vi "Display.vi"(8 "error in":errorcluster, 11 "Input (String) in":refnum<class "Input (String).lvclass">) -> (0 "error out":errorcluster, 3 "Input (String) out":refnum<class "Input (String).lvclass">)   [LabVIEW 2021, in "Pop-Up.lvlib" / "Input (String).lvclass"]
doc: "This vi will display the input pop up waiting for a type String input from the user\n\n<b>Code Developed By:</b>\nDaniel Coons\nTechnology Service Corporation\n1983 S Liberty Drive\nBloomington, IN 47403\nPhone: 812 558-7100\ndaniel.coons@tsc.com\nwww.tsc.com/atcs"
uses:
  Input (String).lvclass
  C:/Development/Open Source/tsc-pop-up/Popup/Popup.lvclass
  Input (String).lvclass/Input (String).ctl
  Popup/Popup.lvclass/Popup.ctl
  Popup/Data Member Access/Read Theme.vi
  Theme/Theme.lvclass
  Popup/Popup.lvclass
  user32.dll
panel:
  out "header":bool
  out "2D Picture":picture
  in  "OK Button":bool
  out "String":string
  in  "Input":string
  out "Input value out":string
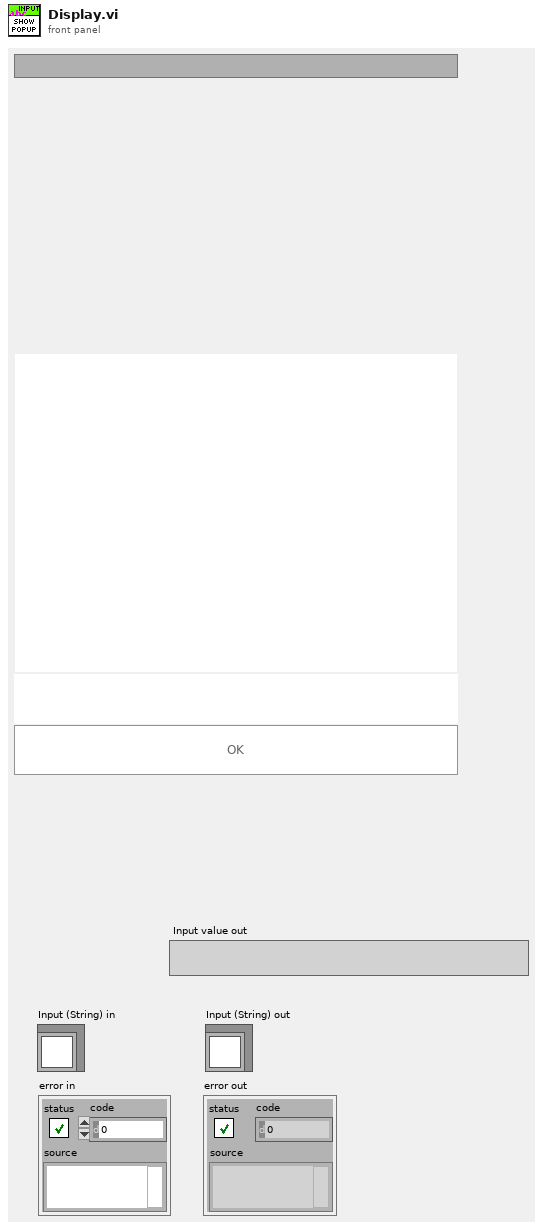
[diagram p1: front panel]
types:
  T1 = typedef "LVPoint32TypeDef.ctl" = cluster{"Horizontal":i32, "Vertical":i32}
  T2 = typedef "LVPositionTypeDef.ctl" = cluster{"Left":i32, "Top":i32}
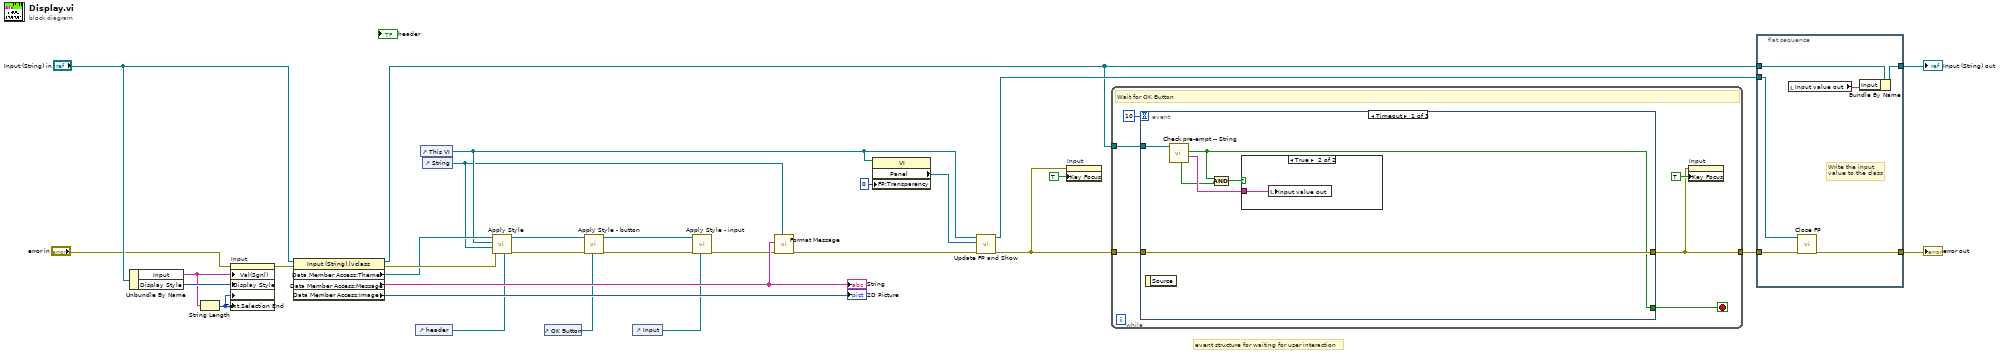
[diagram p0: block diagram]
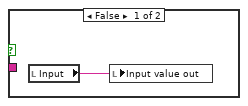
[diagram p2: hidden frame]
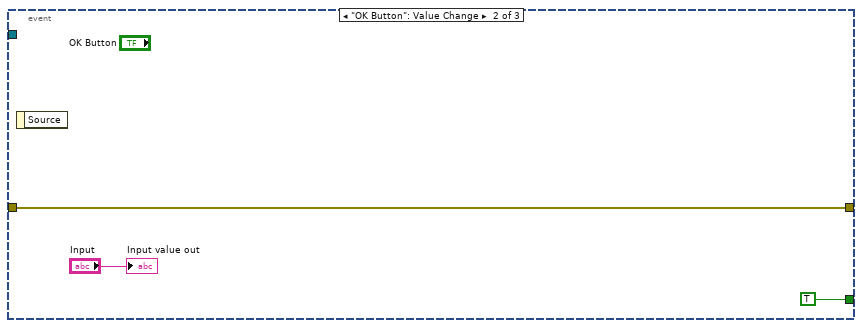
[diagram p3: hidden frame]
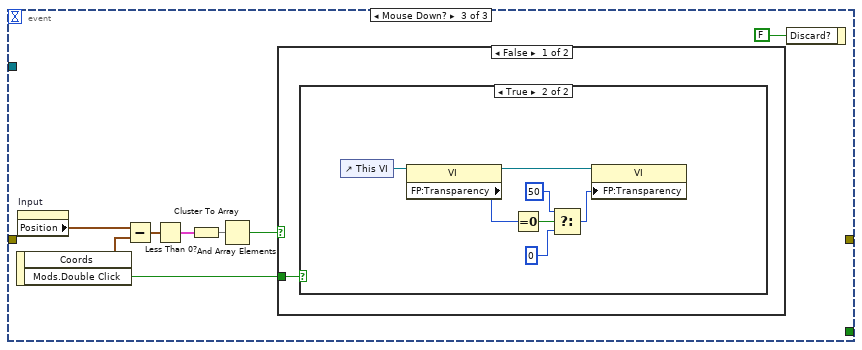
[diagram p4: hidden frame]
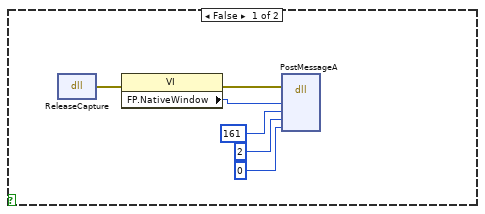
[diagram p5: hidden frame]
diagram:
  # "event structure for waiting for user interaction"
  n1 = Unbundle By Name("Input (String) in") -> ("Input"=w15:string, "Display Style"=w16:u32)
  n2 = String Length(string=w15) -> (length=w14:i32)
  n3 = property on="Input" class="Str"(error in="error in", "Val(Sgnl)"=w15, "Display Style"=w16, "Text.Selection Start"=w14, "Text.Selection End"=w14) -> (error out=w27:errorcluster)  [unwired: 1 in, 1 out]
  n4 = property on="Property Node" class="Input (String).lvclass"(reference="Input (String) in", error in=w27) -> (reference out=w20:refnum<class "Input (String).lvclass">, error out=w26:errorcluster, "Data Member Access:Theme"=w12:refnum<class "Theme.lvclass">, "Data Member Access:Message"=w18:string, "Data Member Access:Image"=→"2D Picture":picture)
  "String" <- w18
  n5 = control-ref of="header"() -> (w9:refnum<vi>)
  n6 = control-ref of="This VI"() -> (w11:refnum<vi>)
  n7 = control-ref of="String"() -> (w10:refnum<vi>)
  n8 = call "Apply Style.vi"("header ref"=w9, "error in"=w26, "message ref"=w10, "pop up ref"=w11, "Theme in"=w12) -> ("error out"=w13:errorcluster, "Theme out"=w5:refnum<class "Theme.lvclass">)  [unwired: 5 in]
  n9 = control-ref of="OK Button"() -> (w4:refnum<vi>)
  n10 = call "Apply Style - button.vi"("button ref"=w4, "error in"=w13, "Theme in"=w5) -> ("error out"=w8:errorcluster, "Theme out"=w6:refnum<class "Theme.lvclass">)  [unwired: 7 in]
  n11 = control-ref of="Input"() -> (w3:refnum<vi>)
  n12 = call "Apply Style - input.vi"("input ref"=w3, "error in (no error)"=w8, "Theme in"=w6) -> ("error out"=w7:errorcluster)  [unwired: 7 in, 1 out]
  n13 = call "Format Message.vi"("formatted string"=w10, "error in"=w7, "String Input"=w18) -> ("error out"=w19:errorcluster)  [unwired: 7 in, 1 out]
  n14 = property on="Property Node" class="VI"(reference=w11, "FP:Transparency"=u8 0 ("Front Panel Window:Transparency")) -> ("Panel"=w24:refnum<vi>)  [unwired: 1 in, 2 out]
  n15 = call "Update FP and Show.vi"("error in (no error)"=w19, "Panel Ref"=w24, "VI in"=w11) -> ("error out"=w21:errorcluster, "VI out"=w23:refnum<vi>)  [unwired: 7 in]
  n16 = property on="Input" class="Str"(error in=w21, "Key Focus"=TRUE) -> ()  [unwired: 1 in, 2 out]
  n17 = while {
    tunnel: w21 -> [w36]
    tunnel: [w31] -> w28
    tunnel: w20 -> [w33]
    stop <- w35 stop-if-true
    # "Wait for OK Button"
    n18 = event shown="[0] Timeout" {
      selector: _ -> [_ _ _]
      dyn-events: _ -> [_ _ _]
      timeout: 10 -> [_ _ _]
      tunnel: w36 -> [w39 w47 _]
      tunnel: [w39 w47 _] -> w31
      tunnel: [w38 TRUE _] -> w35
      tunnel: w33 -> [w37 _ _]
      event Timeout {
        n19 = event-data() -> ()  [unwired: 1 in, 1 out]
        n20 = call "Check pre-empt -- String.vi"("_Popup in"=w37) -> ("Value?"=w42:string, "Pre-empted?"=w38:bool, "Type Match?"=w40:bool)  [unwired: 7 in, 1 out]
        n21 = Compound Arithmetic op=AND(w38, w40) -> (w41:bool)
        n22 = case shown="True" w41 {
          tunnel: w42 -> [_ w44]
          frame False {
            n23 = local read "Input"() -> (w43:string)
            n24 = local write "Input value out"(w43) -> ()
          }
          frame True {
            n25 = local write "Input value out"(w44) -> ()
          }
        }
      }
      event "OK Button": Value Change {
        n26 = event-data() -> ()  [unwired: 1 in, 1 out]
        "Input value out" <- "Input"
      }
      event Mouse Down? {
        n27 = event-data() -> ("Coords"=w50:T1, "Mods.Double Click"=w48:bool)  [unwired: 1 in]
        n28 = property on="Input" class="Str"() -> ("Position"=w54:T2)  [unwired: 2 in, 2 out]
        n29 = Subtract(x=w54, y=w50) -> (x-y=w53:T2)
        n30 = Less Than 0?(x=w53) -> (x < 0?=w52:cluster{"Left":bool, "Top":bool})
        n31 = Cluster To Array(cluster=w52) -> (array=w51:bool[])
        n32 = And Array Elements(Boolean array=w51) -> (logical AND=w49:bool)
        n33 = case shown="False" w49 {
          tunnel: w48 -> [w56 _]
          frame False {
            n34 = case shown="True" w56 {
              frame False {
                n35 = dll-call lib="user32.dll" fn="ReleaseCapture"() -> (error out=w60:errorcluster)  [unwired: 4 in, 1 out]
                n36 = property class="VI"(error in=w60) -> (error out=w61:errorcluster, "FP.NativeWindow"=w62:u64)  [unwired: 1 in, 1 out]
                n37 = dll-call lib="user32.dll" fn="PostMessageA"(error in=w61, "hWnd"=w62, "Msg"=161, "wParam"=2, "lParam"=0) -> ()  [unwired: 7 in, 2 out]
              }
              frame True {
                n38 = control-ref of="This VI"() -> (w69:refnum<vi>)
                n39 = property class="VI"(reference=w69) -> (reference out=w67:refnum<vi>, "FP:Transparency"=w68:u8)  [unwired: 1 in, 1 out]
                n40 = Equal To 0?(x=w68) -> (x = 0?=w66:bool)
                n41 = Select(t=u8 50, s=w66, f=u8 0) -> (s? t:f=w65:u8)
                n42 = property class="VI"(reference=w67, "FP:Transparency"=w65) -> ()  [unwired: 1 in, 2 out]
              }
            }
          }
          frame True {
          }
        }
        n43 = event-data("Discard?"=FALSE) -> ()  [unwired: 1 in, 1 out]
      }
    }
    n44 = property on="Input" class="Str"(error in=w31, "Key Focus"=TRUE) -> ()  [unwired: 1 in, 2 out]
  }
  n45 = flat-sequence {
    tunnel: w28 -> [w75]
    tunnel: [w71] -> w29
    tunnel: w20 -> [w74]
    tunnel: [w73] -> w30
    tunnel: w23 -> [w70]
    frame #0 {
      # "Write the input\nvalue to the class"
      n46 = local read "Input value out"() -> (w72:string)
      n47 = call "Close FP.vi"("error in (no error)"=w75, "VI in"=w70) -> ("error out"=w71:errorcluster)  [unwired: 9 in]
      n48 = Bundle By Name(cluster=w74, "Input"=w72) -> (w73:refnum<class "Input (String).lvclass">)
    }
  }
  "error out" <- w29
  "Input (String) out" <- w30
